vi "SUB_VI_pilotaggio_alimentatore.vi"(8 "Errore ingresso":errorcluster, 9 "Query":string="APPLY P25V,3.3,1.0; OUTP ON; APPL?; ", 10 "Indirizzo":string="04", 11 "byte di lettura":i32=50) -> (0 "Errore in uscita":errorcluster, 1 "Errore in uscita Letto":errorcluster, 2 "Lettura query":string, 3 "Stato scrittura":bool[](array[boolean]), 5 "Stato lettura":bool[](array[boolean]))   [LabVIEW 2023]
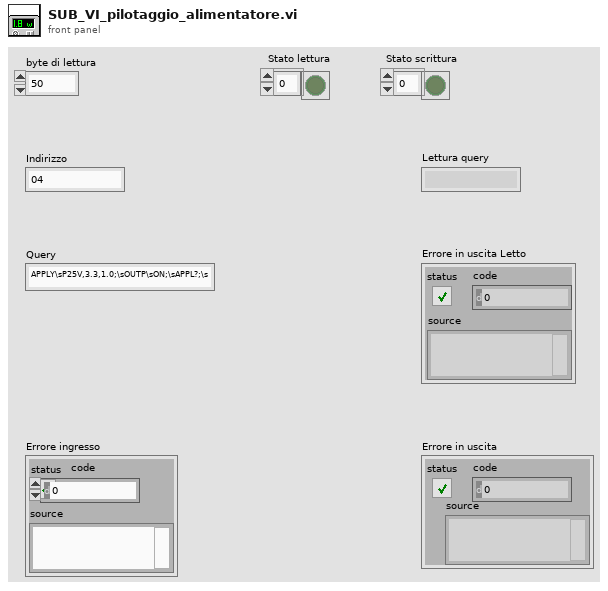
[diagram p1: front panel]
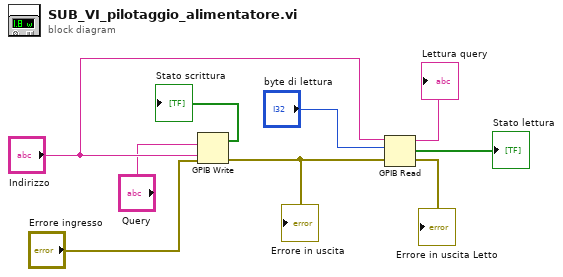
[diagram p0: block diagram]
diagram:
  n1 = GPIB Write(0:"Indirizzo", 1:"Query", 3:"Errore ingresso") -> (5:→"Stato scrittura":bool[], 6:w8:errorcluster)  [unwired: 2 in]
  "Errore in uscita" <- w8
  n2 = GPIB Read(0:"Indirizzo", 1:"byte di lettura", 3:w8) -> (5:→"Lettura query":string, 6:→"Stato lettura":bool[], 7:→"Errore in uscita Letto":errorcluster)  [unwired: 2 in]
